vi "Scott -- strain -- offset plot maker.vi"(11 "Lockin Settings":cluster{"Offset":bool, "GPIB Address":i16}[](array[cluster])) -> (1 "Ok!":bool=TRUE, 2 "appended array":cluster{"data string in":string, bool, bool}[](array[cluster]))   [LabVIEW 2014]
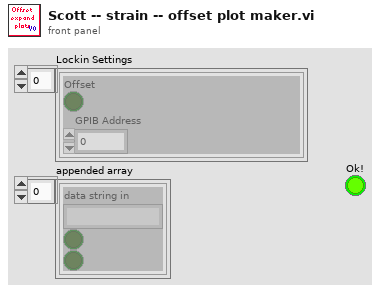
[diagram p1: front panel]
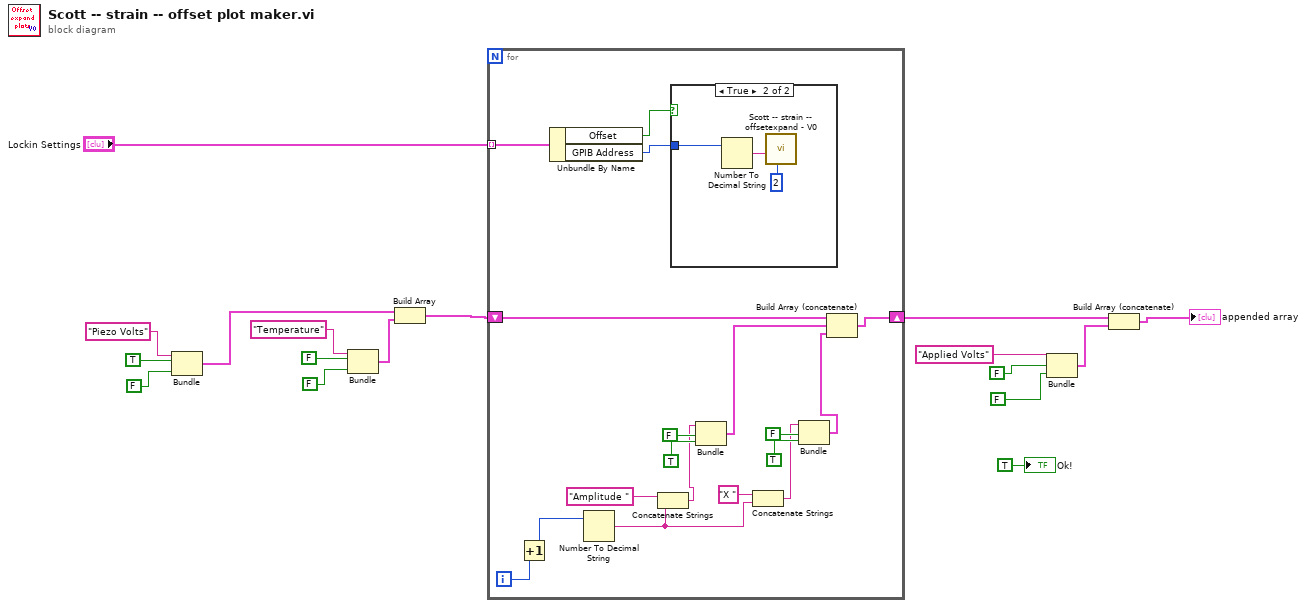
[diagram p0: block diagram]
diagram:
  n1 = Bundle("data string in"="Piezo Volts", TRUE, FALSE) -> (w3:cluster{"data string in":string, bool, bool})  [unwired: 1 in]
  n2 = Bundle("data string in"="Temperature", FALSE, FALSE) -> (w2:cluster{"data string in":string, bool, bool})  [unwired: 1 in]
  n3 = Build Array(w3, w2) -> (w16:cluster{"data string in":string, bool, bool}[])
  n4 = for {
    tunnel: "Lockin Settings" -> [w35] mode=indexing
    shift-right: [w19] -> w12
    shift-left: w16 -> [w28]
    i -> [w29]
    n5 = Increment(x=w29) -> (x+1=w18:i32)
    n6 = Unbundle By Name(w35) -> ("Offset"=w34:bool, "GPIB Address"=w33:i16)
    n7 = Number To Decimal String(number=w18) -> (decimal integer string=w30:string)  [unwired: 1 in]
    n8 = Concatenate Strings("Amplitude " ("data string in"), w30) -> (w23:string)
    n9 = case shown="True" w34 {
      tunnel: w33 -> [_ w36]
      frame False {
      }
      frame True {
        n10 = Number To Decimal String(number=w36) -> (decimal integer string=w38:string)  [unwired: 1 in]
        n11 = call "Scott -- strain -- offsetexpand - V0.vi"("offset expand, 1 for 10, 2 for 100"=i64 2, "address string"=w38) -> ()  [unwired: 9 in, 1 out]
      }
    }
    n12 = Bundle(w23, FALSE, TRUE) -> (w21:cluster{string, bool, bool})  [unwired: 1 in]
    n13 = Concatenate Strings("X " ("data string in"), w30) -> (w22:string)
    n14 = Bundle(w22, FALSE, TRUE) -> (w20:cluster{string, bool, bool})  [unwired: 1 in]
    n15 = Build Array (concatenate)(w28, w21, w20) -> (w19:cluster{"data string in":string, bool, bool}[])
  }
  n16 = Bundle("data string in"="Applied Volts", FALSE, FALSE) -> (w11:cluster{"data string in":string, bool, bool})  [unwired: 1 in]
  n17 = Build Array (concatenate)(w12, w11) -> (→"appended array":cluster{"data string in":string, bool, bool}[])
  "Ok!" <- TRUE
